vi "VisualInspectionAHUold.vi"(8 "error in (no error)":errorcluster, 11 "TableRef":refnum<vi>) -> (0 "error out":errorcluster, 2 "VisualInspectionResult":bool)   [LabVIEW 2017]
panel:
  in  "7.3 2":bool
  in  "Cancel Button":bool
  in  "OK Button":bool
  in  "7.5.1.1":bool
  in  "7.3":bool
  in  "7.2.3":bool
  in  "7.2.4":bool
  in  "7.2.5":bool
  in  "6.2.2.1":bool
  in  "6.2.2.2":bool
  in  "6.2.2.3":bool
  in  "6.2.2.4":bool
  in  "7.1":bool
  in  "6.2.1.1":bool
  in  "7.2.2":bool
  in  "6.1.2":bool
  in  "7.2.1.1":bool
  in  "7.2.1":bool
  in  "6.1.1":bool
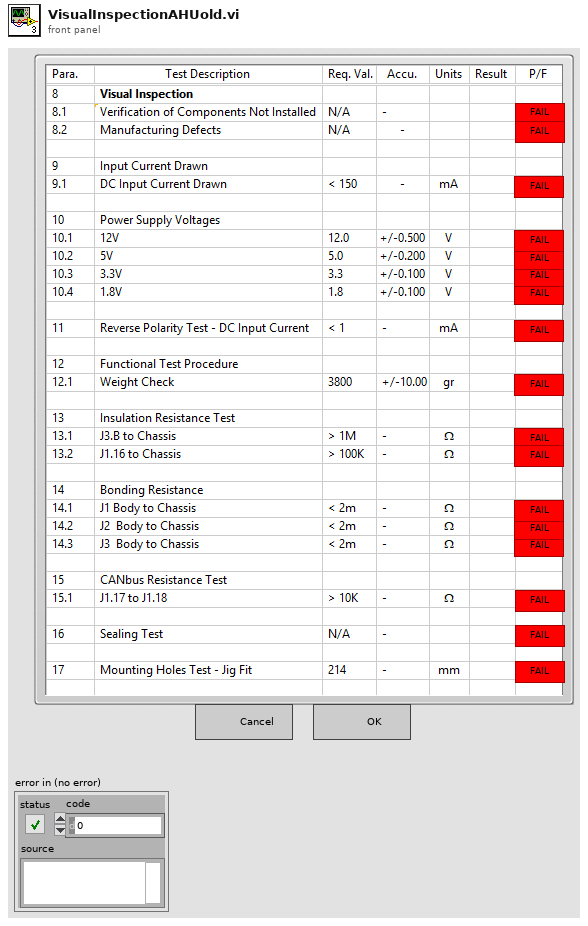
[diagram p1: front panel]
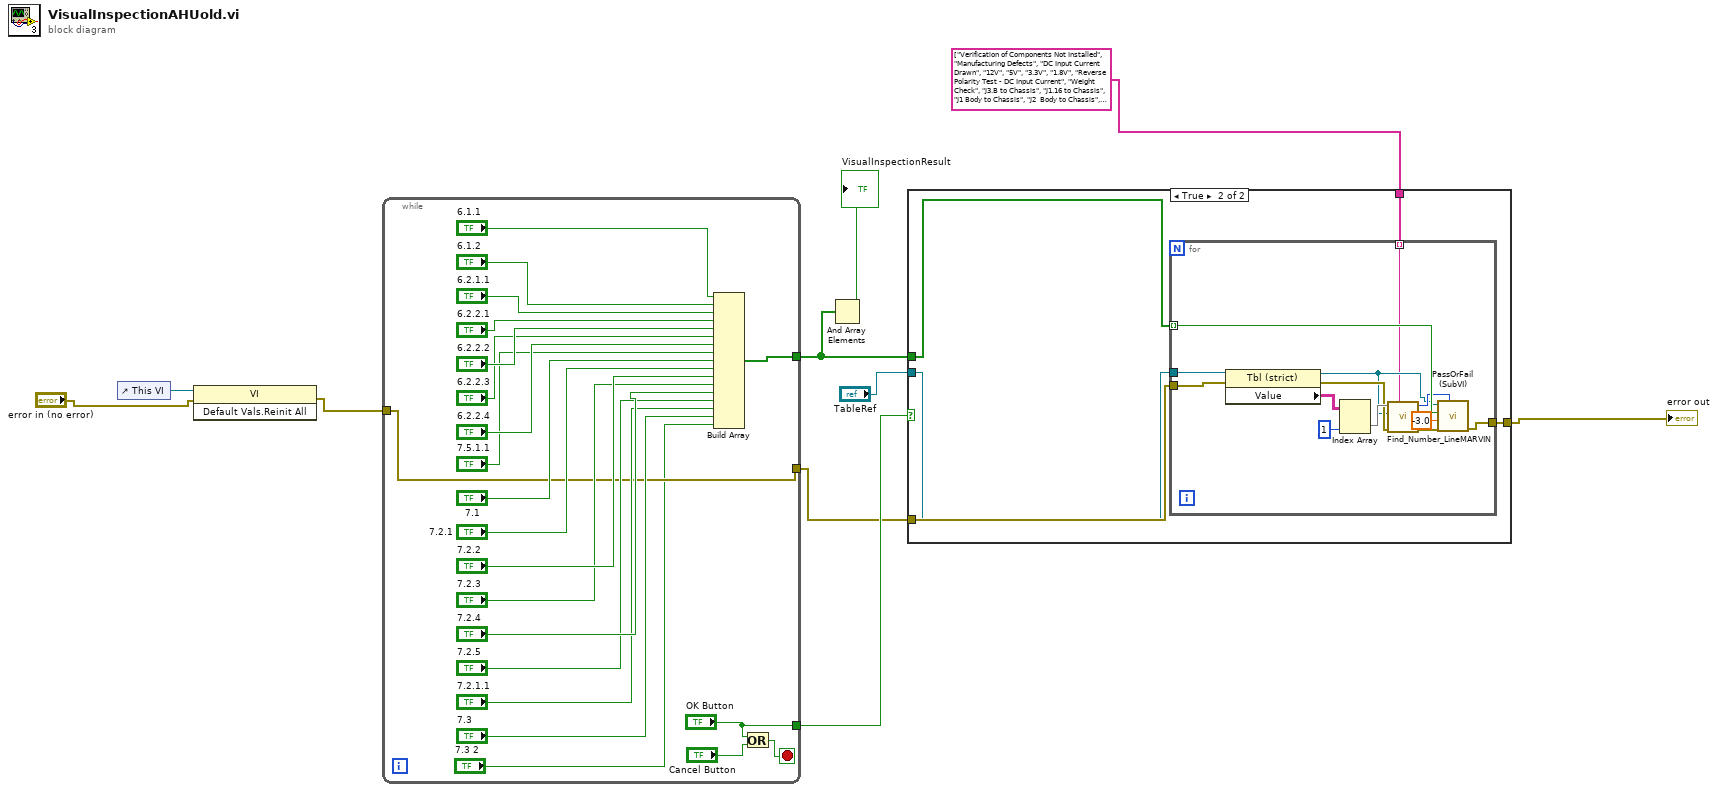
[diagram p0: block diagram]
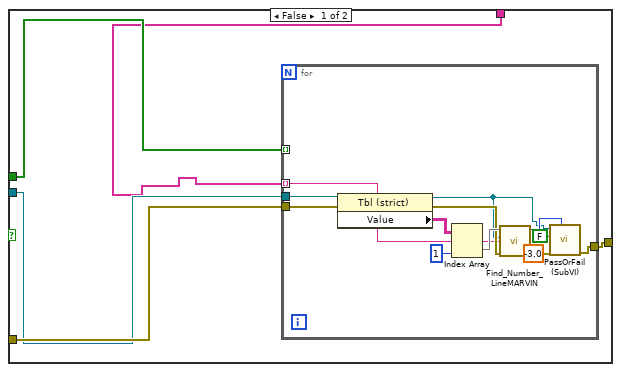
[diagram p2: hidden frame]
diagram:
  n1 = control-ref of="This VI"() -> (w6:refnum<vi>)
  n2 = invoke class="VI" method="Default Vals.Reinit All"(reference=w6, error in="error in (no error)") -> (error out=w10:errorcluster)  [unwired: 1 in, 2 out]
  n3 = while {
    tunnel: w10 -> [w13]
    tunnel: [w15] -> w3
    tunnel: ["OK Button"] -> w9
    tunnel: [w13] -> w8
    stop <- w31 stop-if-true
    n4 = Build Array("6.1.1", "6.1.2", "6.2.1.1", "6.2.2.1", "6.2.2.2", "6.2.2.3", "6.2.2.4", "7.5.1.1", "7.1", "7.2.1", "7.2.2", "7.2.3", "7.2.4", "7.2.5", "7.2.1.1", "7.3", "7.3 2") -> (w15:bool[])
    n5 = Or(x="OK Button", y="Cancel Button") -> (x .or. y?=w31:bool)
  }
  n6 = And Array Elements(Boolean array=w3) -> (logical AND=→"VisualInspectionResult":bool)
  n7 = case shown="True" w9 {
    tunnel: w3 -> [w37 w55]
    tunnel: w8 -> [w36 w54]
    tunnel: [w35 w53] -> w4
    tunnel: "TableRef" -> [w34 w52]
    tunnel: string[] ["Verification of Components Not Installed", "Manufacturing Defects", "DC Input Current Drawn", "12V", "5V", "3.3V", "1.8V", "Reverse Polarity Test - DC Input Current", "Weight Check", "J3.B to Chassis", "J1.16 to Chassis", "J1 Body to Chassis", "J2  Body to Chassis", "J3  Body to Chassis", "J1.17 to J1.18", "Sealing Test", "Mounting Holes Test - Jig Fit"] ("deleted portion 3") -> [w33 w51]
    frame False {
      n8 = for {
        tunnel: w33 -> [w46] mode=indexing
        tunnel: w37 -> [_] mode=indexing
        tunnel: w36 -> [w43]
        tunnel: [w42] -> w35
        tunnel: w34 -> [w41]
        n9 = property class="Tbl (strict)"(reference=w41, error in=w43) -> (reference out=w38:refnum<vi>, error out=w47:errorcluster, "Value"=w50:string[][])
        n10 = Index Array(array=w50, index (col)=1 ("disabled index (col)")) -> (element=w48:string[])  [unwired: 1 in]
        n11 = call "Find_Number_LineMARVIN.vi"("Test Paragraph"=w46, "error in"=w47, "TableIn"=w38, "Row Headers[]"=w48) -> ("error out"=w45:errorcluster, "Line number"=w44:i32)  [unwired: 1 in, 2 out]
        n12 = call "PassOrFail (SubVI).vi"("index (row)"=w44, "error in (no error)"=w45, "Data in"=-3.0, "Pass?Fail"=FALSE ("Boolean"), "Table in"=w38) -> ("error out"=w42:errorcluster)  [unwired: 6 in]
      }
    }
    frame True {
      n13 = for {
        tunnel: w55 -> [w63] mode=indexing
        tunnel: w54 -> [w61]
        tunnel: [w60] -> w53
        tunnel: w52 -> [w59]
        tunnel: w51 -> [w56] mode=indexing
        n14 = property class="Tbl (strict)"(reference=w59, error in=w61) -> (reference out=w57:refnum<vi>, error out=w65:errorcluster, "Value"=w68:string[][])
        n15 = Index Array(array=w68, index (col)=1 ("disabled index (col)")) -> (element=w66:string[])  [unwired: 1 in]
        n16 = call "Find_Number_LineMARVIN.vi"("Test Paragraph"=w56, "error in"=w65, "TableIn"=w57, "Row Headers[]"=w66) -> ("error out"=w64:errorcluster, "Line number"=w62:i32)  [unwired: 1 in, 2 out]
        n17 = call "PassOrFail (SubVI).vi"("index (row)"=w62, "error in (no error)"=w64, "Data in"=-3.0, "Pass?Fail"=w63, "Table in"=w57) -> ("error out"=w60:errorcluster)  [unwired: 6 in]
      }
    }
  }
  "error out" <- w4
